vi "GDSProject_GetTargetClasses.vi"(6 "ExcludeBuilds(Yes)":bool=TRUE, 8 "error in (no error)":errorcluster, 9 "ExcludeTargets(Yes)":bool=TRUE, 10 "ExcludeDependencies(No)":bool, 11 "TargetItem in":refnum<vi>) -> (0 "error out":errorcluster, 1 "LvInterfaces":refnum<vi>[](array[refnum]), 2 "LvClasses":refnum<vi>[](array[refnum]), 3 "TargetItem out":refnum<vi>, 4 "LvInterfaces(Path)":path[](array[path]), 5 "LvClasses(Path)":path[](array[path]))   [LabVIEW 2020]
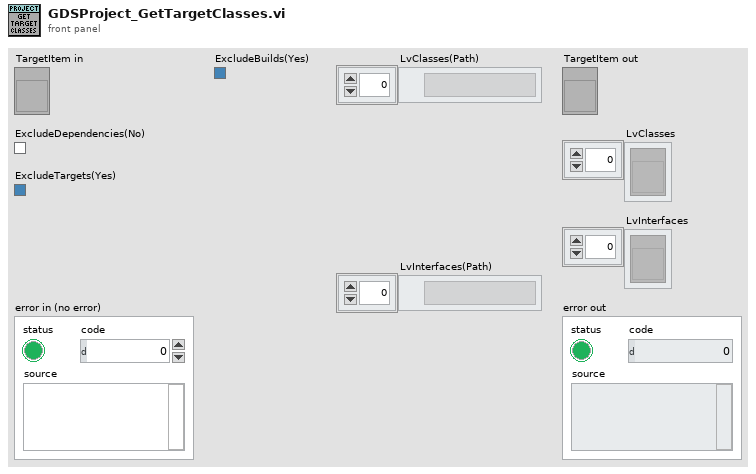
[diagram p1: front panel]
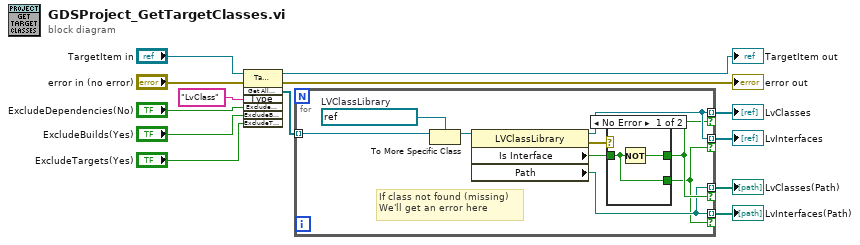
[diagram p0: block diagram]
diagram:
  n1 = invoke class="TargetItem" method="Get All Descendents"(reference="TargetItem in", error in="error in (no error)", "Type"="LvClass", "Exclude Dependencies"="ExcludeDependencies(No)", "ExcludeBuilds"="ExcludeBuilds(Yes)", "ExcludeTargets"="ExcludeTargets(Yes)") -> (reference out=→"TargetItem out":refnum<vi>, error out=→"error out":errorcluster, "All Descendents"=w6:refnum<vi>[])  [unwired: 1 in, 4 out]
  n2 = for {
    tunnel: w6 -> [w22] mode=indexing
    tunnel: [w19] -> w4 mode=indexing if=w18
    tunnel: [w19] -> w5 mode=indexing if=w14
    tunnel: [w17] -> w2 mode=indexing if=w18
    tunnel: [w17] -> w1 mode=indexing if=w14
    w21 = refnum<vi> refnum  # LVClassLibrary
    # "If class not found (missing)\nWe'll get an error here"
    n3 = To More Specific Class(target class=w21, reference=w22) -> (specific class reference=w20:refnum<vi>)  [unwired: 1 in, 1 out]
    n4 = property class="LVClassLibrary"(reference=w20) -> (reference out=w19:refnum<vi>, error out=w16:errorcluster, "Is Interface"=w15:bool, "Path"=w17:path)  [unwired: 1 in]
    n5 = case shown="No Error" w16 {
      tunnel: [w24 _] -> w18
      tunnel: w15 -> [w23 _]
      tunnel: [w23 _] -> w14
      frame No Error {
        n6 = Not(x=w23) -> (.not. x?=w24:bool)
      }
      frame Error {
      }
    }
  }
  "LvClasses" <- w4
  "LvInterfaces" <- w5
  "LvInterfaces(Path)" <- w1
  "LvClasses(Path)" <- w2
